vi "Sub_CalculateScaledDistance.vi"(1 "Width scaling":dbl=1.0, 2 "Height scaling":dbl=1.0, 3 "Width iteration":i32, 4 "Height iteration":i32, 5 "Object width":u8, 6 "Object height":u8) -> (0 "Scaled distance":dbl)   [LabVIEW 2021]
panel:
  # "Inputs:"
  # "Outputs:"
  # "Required:"
  # "Optional:"
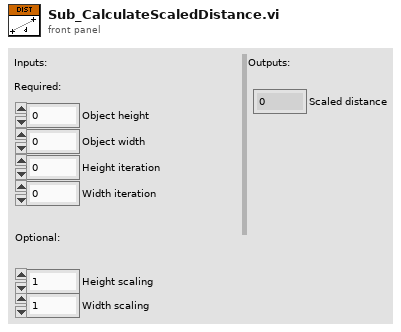
[diagram p1: front panel]
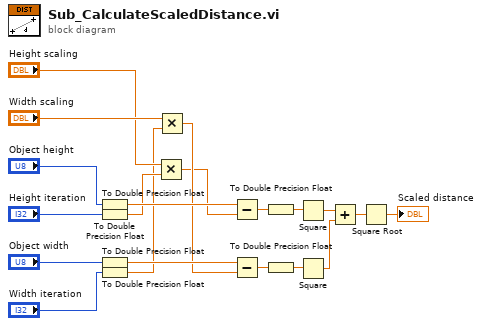
[diagram p0: block diagram]
diagram:
  n1 = To Double Precision Float(number="Object height") -> (double precision float=w6:dbl)
  n2 = To Double Precision Float(number="Height iteration") -> (double precision float=w4:dbl)
  n3 = To Double Precision Float(number="Object width") -> (double precision float=w8:dbl)
  n4 = To Double Precision Float(number="Width iteration") -> (double precision float=w3:dbl)
  n5 = Multiply(x="Height scaling", y=w4) -> (x*y=w1:dbl)
  n6 = Multiply(x="Width scaling", y=w3) -> (x*y=w2:dbl)
  n7 = Subtract(x=w6, y=w1) -> (x-y=w10:dbl)
  n8 = Subtract(x=w8, y=w2) -> (x-y=w13:dbl)
  n9 = To Double Precision Float(number=w10) -> (double precision float=w11:dbl)
  n10 = To Double Precision Float(number=w13) -> (double precision float=w12:dbl)
  n11 = Square(x=w11) -> (x^2=w16:dbl)
  n12 = Square(x=w12) -> (x^2=w15:dbl)
  n13 = Add(x=w16, y=w15) -> (x+y=w17:dbl)
  n14 = Square Root(x=w17) -> (sqrt(x)=→"Scaled distance":dbl)
